vi "Simulate_Power_Supply.vi"(8 "Time to run current [ms]":u32, 11 "Current [A]":dbl) -> (0 "Time indicator [ms]":u32, 3 "Current Indicator [A]":dbl)   [LabVIEW 2019]
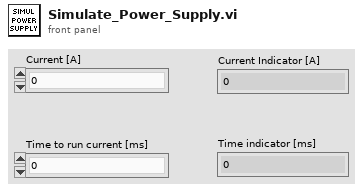
[diagram p1: front panel]
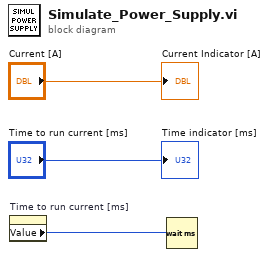
[diagram p0: block diagram]
diagram:
  n1 = property on="Time to run current [ms]" class="DigNum (strict)"() -> ("Value"=w3:u32)  [unwired: 2 in, 2 out]
  n2 = Wait (ms)(milliseconds to wait=w3) -> ()  [unwired: 1 out]
  "Current Indicator [A]" <- "Current [A]"
  "Time indicator [ms]" <- "Time to run current [ms]"
